vi "save_target.vi"   [LabVIEW 2011]
doc: "Save data form daq loop"
uses:
  controls.llb/RTFIFO name.ctl
  controls.llb/RTFIFO operate.ctl
types:
  T1 = typedef "RTFIFO operate.ctl" = enum16{"Creat", "Write", "Read", "Delete"}
  T2 = typedef "RTFIFO name.ctl" = enum16{"command_daq", "command_control", "data for save", "data for host", "dev status", "status for save"}
  T3 = typedef "data from RTFIFO.ctl" = cluster{"data for save":dbl[][], "data for host":dbl[][], "command_daq":u16, "command_control":u16, "dev status":u16[][], "status for save":u16[][]}
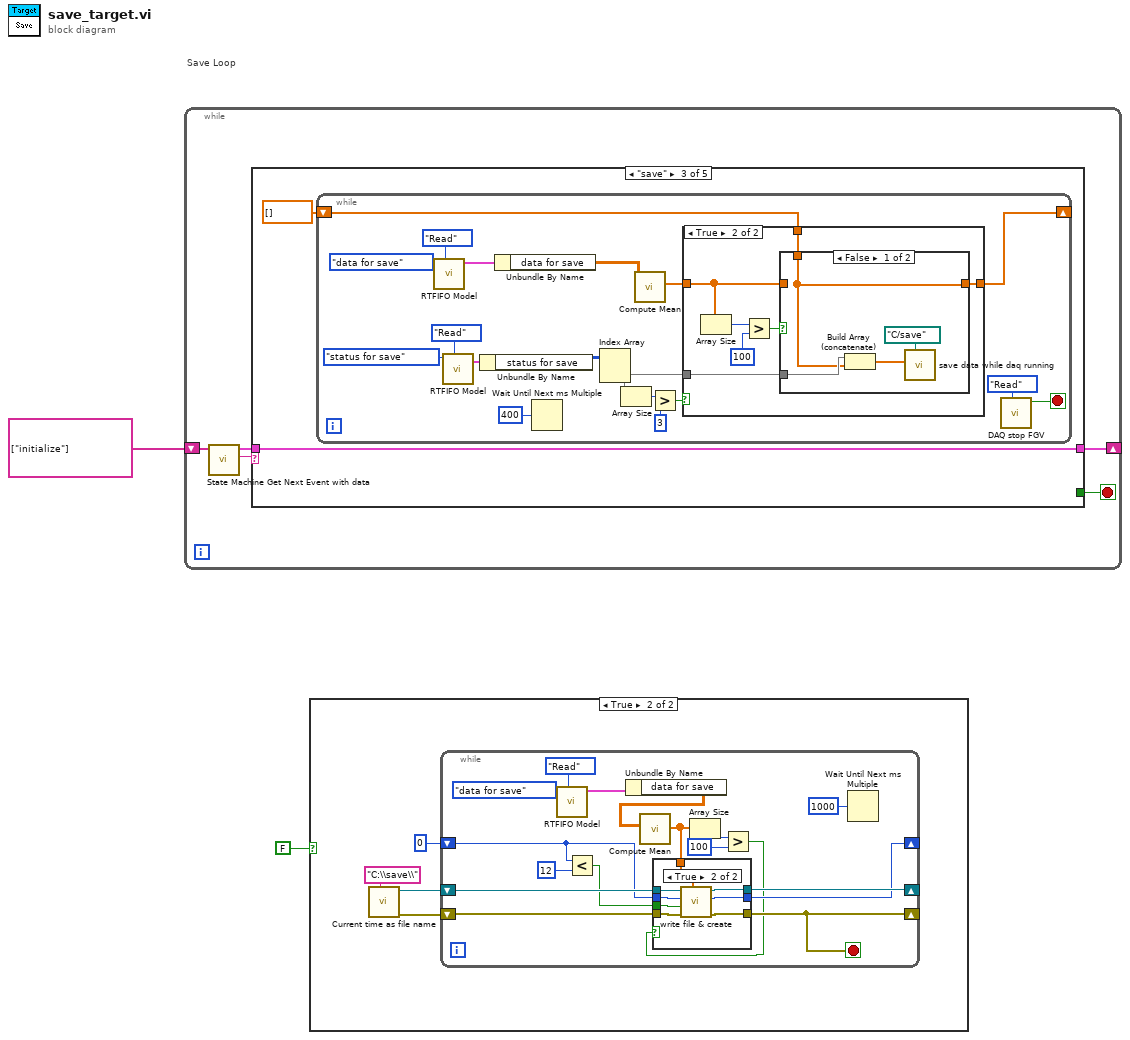
[diagram p0: block diagram]
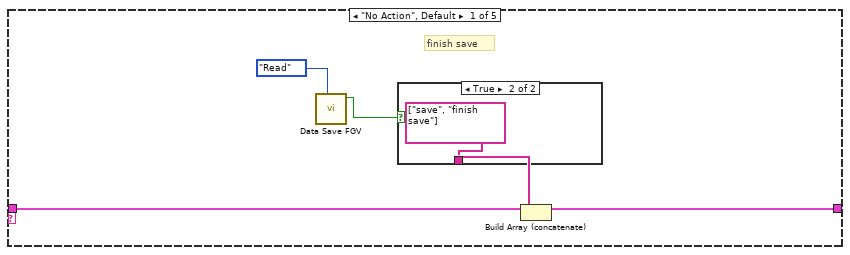
[diagram p4: hidden frame]
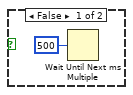
[diagram p5: hidden frame]
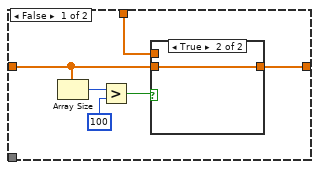
[diagram p7: hidden frame]
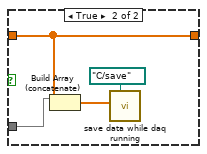
[diagram p9: hidden frame]
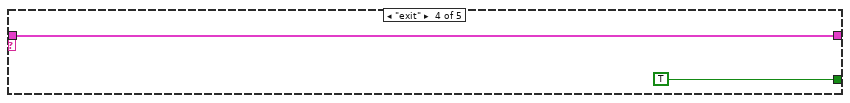
[diagram p10: hidden frame]
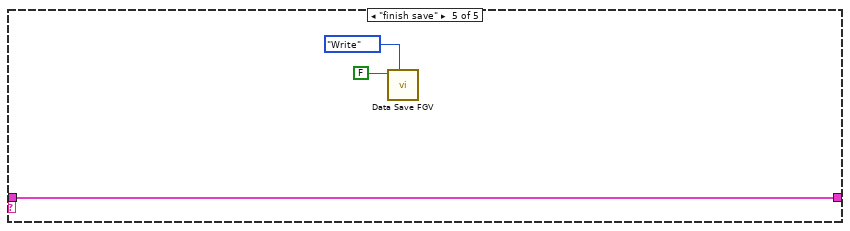
[diagram p11: hidden frame]
diagram:
  # "Save Loop"
  n1 = while {
    shift-right: [w4] -> _
    shift-left: string[] ["initialize"] -> [w7]
    stop <- w3 stop-if-true
    n2 = call "State Machine Get Next Event with data.vi"("enent data queue in"=w7) -> ("next event"=w6:string, "event queue out"=w5:cluster{"event":string, "data":string}[])  [unwired: 5 in]
    n3 = case shown="\"save\"" w6 {
      tunnel: w5 -> [w12 w15 w17 w60 w61]
      tunnel: [w11 w15 w17 w60 w61] -> w4
      tunnel: [_ _ _ TRUE _] -> w3
      frame "No Action", Default {
        # "finish save"
        n4 = call "Data Save FGV .vi"("W/R"=enum16{"Read", "Write"}."Read") -> ("Save"=w9:bool)  [unwired: 10 in]
        n5 = case shown="True" w9 {
          tunnel: [_ string[] ["save", "finish save"]] -> w8
          frame False {
            n6 = Wait Until Next ms Multiple(millisecond multiple=u32 500) -> ()  [unwired: 1 out]
          }
          frame True {
          }
        }
        n7 = Build Array (concatenate)(w12, w8) -> (w11:cluster{"event":string, "data":string}[])
      }
      frame "initialize" {
      }
      frame "save" {
        n8 = while {
          shift-right: [w19] -> _
          shift-left: dbl[] [] ("data") -> [w18]
          stop <- w29 stop-if-true
          n9 = call "RTFIFO Model.vi"("operate"=RTFIFO_operate."Read", "FIFO name"=RTFIFO_name."data for save") -> ("data"=w34:T3)  [unwired: 8 in, 1 out]
          n10 = call "RTFIFO Model.vi"("operate"=RTFIFO_operate."Read", "FIFO name"=RTFIFO_name."status for save") -> ("data"=w26:T3)  [unwired: 8 in, 1 out]
          n11 = Unbundle By Name(w26) -> ("status for save"=w25:u16[][])
          n12 = Unbundle By Name(w34) -> ("data for save"=w35:dbl[][])
          n13 = Wait Until Next ms Multiple(millisecond multiple=u32 400) -> ()  [unwired: 1 out]
          n14 = Index Array(array=w25) -> (element=w20:u16[])  [unwired: 2 in]
          n15 = Array Size(array=w20) -> (size(s)=w24:i32)
          n16 = call "Compute Mean.vi"("2D array"=w35) -> ("data"=w21:dbl[])  [unwired: 10 in]
          n17 = Greater?(x=w24, y=3) -> (0:w22:bool)
          n18 = case shown="True" w22 {
            tunnel: w21 -> [w38 w46]
            tunnel: w20 -> [_ w47]
            tunnel: [w37 w45] -> w19
            tunnel: w18 -> [w36 w44]
            frame False {
              n19 = Array Size(array=w38) -> (size(s)=w41:i32)
              n20 = Greater?(x=w41, y=100) -> (0:w39:bool)
              n21 = case shown="True" w39 {
                tunnel: w38 -> [_ w43]
                tunnel: [w42 w43] -> w37
                tunnel: w36 -> [w42 _]
                frame False {
                }
                frame True {
                }
              }
            }
            frame True {
              n22 = Array Size(array=w46) -> (size(s)=w50:i32)
              n23 = Greater?(x=w50, y=100) -> (0:w48:bool)
              n24 = case shown="False" w48 {
                tunnel: w47 -> [w52 w57]
                tunnel: w46 -> [_ w55]
                tunnel: [w51 w55] -> w45
                tunnel: w44 -> [w51 _]
                frame False {
                  n25 = Build Array (concatenate)(w52, w51) -> (w53:dbl[])
                  n26 = call "save data while daq running.vi"("test status and data"=w53, "file path"=path "C:/save") -> ()  [unwired: 9 in, 1 out]
                }
                frame True {
                  n27 = Build Array (concatenate)(w57, w55) -> (w56:dbl[])
                  n28 = call "save data while daq running.vi"("test status and data"=w56, "file path"=path "C:/save") -> ()  [unwired: 9 in, 1 out]
                }
              }
            }
          }
          n29 = call "DAQ stop FGV.vi"("W/R"=enum16{"Read", "Write"}."Read") -> ("stop ?"=w29:bool)  [unwired: 10 in]
        }
      }
      frame "exit" {
      }
      frame "finish save" {
        n30 = call "Data Save FGV .vi"("W/R"=enum16{"Read", "Write"}."Write", "Save?"=FALSE) -> ()  [unwired: 9 in, 1 out]
      }
    }
  }
  n31 = case shown="True" FALSE {
    frame False {
    }
    frame True {
      n32 = call "Current time as file name.vi"("string"="C:\\save\\") -> ("error out"=w65:errorcluster, "refnum out"=w66:refnum<file>)  [unwired: 9 in]
      n33 = while {
        shift-right: [w75] -> _
        shift-left: w66 -> [w80]
        shift-right: [w73] -> _
        shift-left: w65 -> [w76]
        shift-right: [w74] -> _
        shift-left: 0 -> [w79]
        stop <- w73 stop-if-true
        n34 = call "RTFIFO Model.vi"("operate"=RTFIFO_operate."Read", "FIFO name"=RTFIFO_name."data for save") -> ("data"=w82:T3)  [unwired: 8 in, 1 out]
        n35 = Less?(x=w79, y=12) -> (x < y?=w77:bool)
        n36 = Unbundle By Name(w82) -> ("data for save"=w81:dbl[][])
        n37 = call "Compute Mean.vi"("2D array"=w81) -> ("data"=w69:dbl[])  [unwired: 10 in]
        n38 = Array Size(array=w69) -> (size(s)=w72:i32)
        n39 = Greater?(x=w72, y=100) -> (0:w70:bool)
        n40 = case shown="True" w70 {
          tunnel: w80 -> [w87 w95]
          tunnel: w79 -> [w85 w94]
          tunnel: w77 -> [_ w93]
          tunnel: w76 -> [w86 w92]
          tunnel: [w87 w91] -> w75
          tunnel: [w85 w90] -> w74
          tunnel: [w86 w89] -> w73
          tunnel: w69 -> [_ w88]
          frame False {
          }
          frame True {
            n41 = call "write file & create.vi"("Array"=w88, "error in"=w92, "Boolean"=w93, "Numeric"=w94, "refnum in"=w95) -> ("error out 2"=w89:errorcluster, "Numeric 2"=w90:i32, "file refnum"=w91:refnum<file>)  [unwired: 2 in]
          }
        }
        n42 = Wait Until Next ms Multiple(millisecond multiple=u32 1000) -> ()  [unwired: 1 out]
      }
    }
  }
